vi "Fetch Limit Fails.vi"(8 "error in (no error)":errorcluster, 9 "Measurement Number (1: Measurement 1)":u32(ring)=1 items=["Measurement 1"=1, "Measurement 2"=2, "Measurement 3"=3, "Measurement 4"=4], 10 "Maximum Time (30000 ms)":u32=30000, 11 "VISA resource name":refnum<visa-resource-name>) -> (0 "error out":errorcluster, 1 "Limit Test Pass?":bool=TRUE, 2 "Limit Failure Count":u32, 3 "VISA resource name out":refnum<visa-resource-name>)   [LabVIEW 2011, in "Agilent N432A.lvlib"]
doc: "Returns the limit test result, including whether there have been any limit failures and the total number of limit failures for the specified window/measurement. You need to initiate an acquisition with the Initiate VI prior to calling this VI.\n\n<B>Note:</B> \n\nUse this VI only with other low-level VIs. The high-level VIs automatically incorporate this functionality. This VI does not check the instrument status."
uses:
  <instrlib>/Agilent N432A/Agilent N432A.lvlib
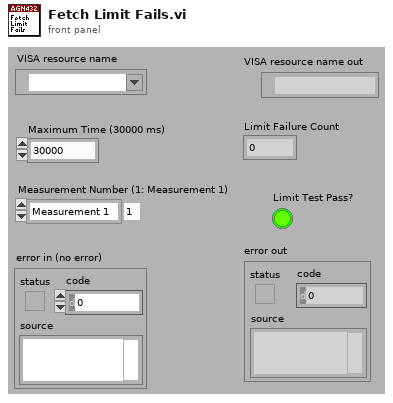
[diagram p1: front panel]
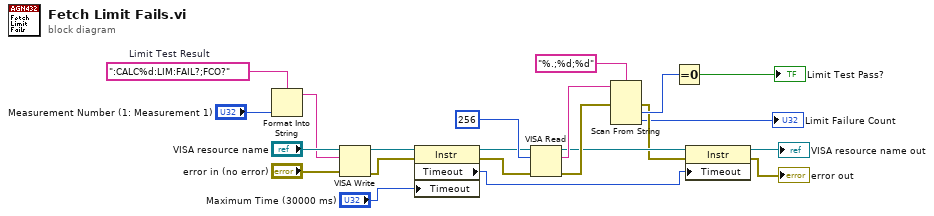
[diagram p0: block diagram]
diagram:
  w16 = ":CALC%d:LIM:FAIL?;FCO?"  # Limit Test Result
  n1 = Format Into String(format string=w16, "Measurement Number (1: Measurement 1)") -> (resulting string=w15:string)  [unwired: 2 in, 1 out]
  n2 = VISA Write(VISA resource name="VISA resource name", write buffer=w15, error in (no error)="error in (no error)") -> (VISA resource name out=w11:refnum<visa-resource-name>, error out=w10:errorcluster)  [unwired: 1 out]
  n3 = property class="Instr"(reference=w11, error in=w10, "Timeout"="Maximum Time (30000 ms)") -> (reference out=w9:refnum<visa-resource-name>, error out=w8:errorcluster, "Timeout"=w12:u32)
  n4 = VISA Read(VISA resource name=w9, byte count=u32 256, error in (no error)=w8) -> (VISA resource name out=w6:refnum<visa-resource-name>, read buffer=w21:string, error out=w19:errorcluster)  [unwired: 1 out]
  n5 = Scan From String(format string="%.;%d;%d", input string=w21, error in=w19) -> (error out=w5:errorcluster, output 1=w13:i32, output 2=→"Limit Failure Count":u32)  [unwired: 3 in, 2 out]
  n6 = Equal To 0?(x=w13) -> (x = 0?=→"Limit Test Pass?":bool)
  n7 = property class="Instr"(reference=w6, error in=w5, "Timeout"=w12) -> (reference out=→"VISA resource name out":refnum<visa-resource-name>, error out=→"error out":errorcluster)
